vi "MRC Read.vi"(8 "error in (no error)":errorcluster, 9 "Message Data":variant, 11 "Data  in":T1={"MFC Definition"={"MFC Port"="", "MFC Enable"=TRUE, "Baud Rate"=0, "Interface type"=enum."RS-485", "Address"=0}, "Set Point Options"={"Setpoint Value"=0.0, "Mass Flow EU 2"="", "Setpoint Source"="", "Valve Mode"=""}, "Writer Queue"=refnum, "Enable"=FALSE, "Update Rate"=0, "MRC Chamber Enable"=FALSE, "Selected Gas"="", "Address String"=""} {"Set Point Options"."Setpoint Value" min=0.0 max=0.62495 format="%.5f"}) -> (0 "error out":errorcluster, 1 "Message Data Out":variant, 2 "Error Message":variant, 3 "Data out":T1={"MFC Definition"={"MFC Port"="", "MFC Enable"=TRUE, "Baud Rate"=0, "Interface type"=enum."RS-485", "Address"=0}, "Set Point Options"={"Setpoint Value"=0.0, "Mass Flow EU 2"="", "Setpoint Source"="", "Valve Mode"=""}, "Writer Queue"=refnum, "Enable"=FALSE, "Update Rate"=0, "MRC Chamber Enable"=FALSE, "Selected Gas"="", "Address String"=""} {"Set Point Options"."Setpoint Value" min=0.0 max=0.62495 format="%.5f"})   [LabVIEW 2020, in "MRC Module.lvlib"]
doc: "Perform the acquisition. Replace the contents of this diagram with calls to acquisition hardware."
uses:
  MRC Module.lvlib
  MRC Configuration.ctl
  support/Message Queue/Message Cluster.ctl
  support/Message Queue/Message Queue.lvlib
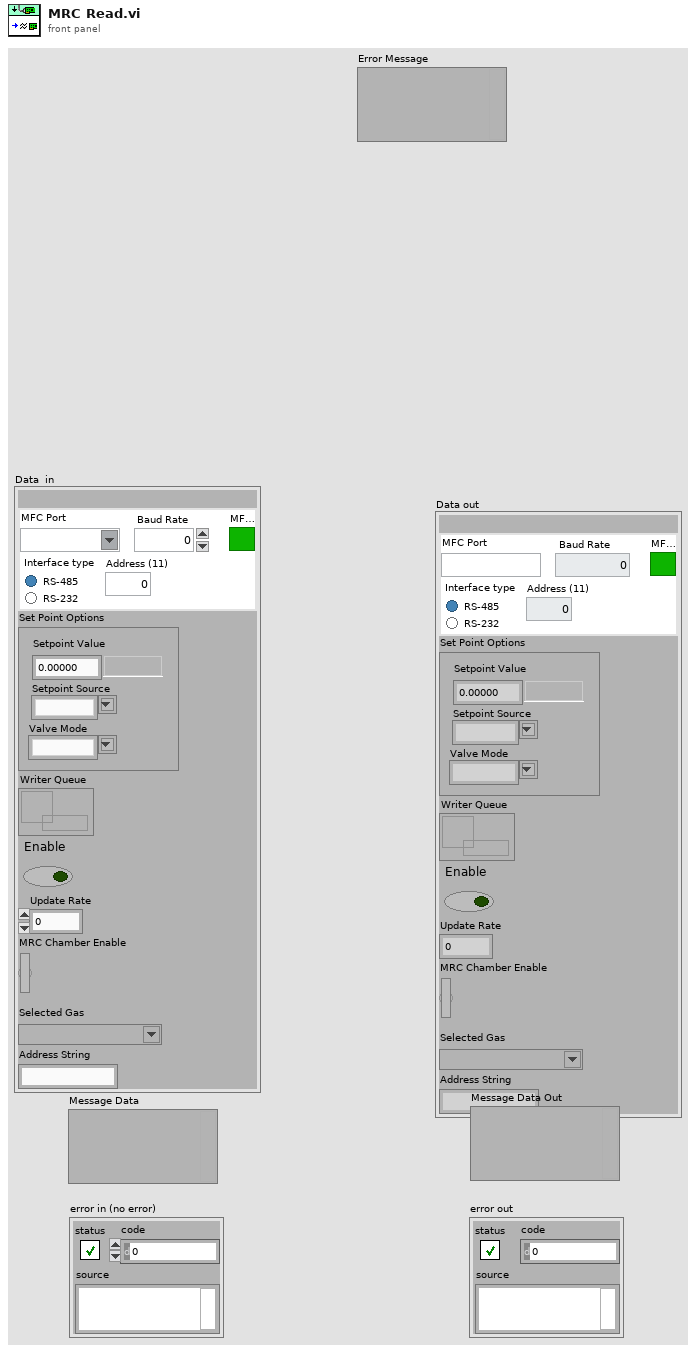
[diagram p1: front panel]
types:
  T1 = typedef "MRC Module.lvlib/MRC Configuration.ctl" = cluster{"MFC Definition":cluster{"MFC Port":refnum<visa-resource-name>, "MFC Enable":bool, "Baud Rate":i32, "Interface type":enum32{"RS-485", "RS-232"}, "Address":i32}, "Set Point Options":cluster{"Setpoint Value":dbl, "Mass Flow EU 2":string, "Setpoint Source":string, "Valve Mode":string}, "Writer Queue":refnum<queue>, "Enable":bool, "Update Rate":u32, "MRC Chamber Enable":bool, "Selected Gas":string, "Address String":string}
  T2 = typedef "Message Queue.lvlib/Message Cluster.ctl" = cluster{"Message":string, "Message Data":variant}
  T3 = cluster{"string array[0]":string, "string array[1]":string, "string array[2]":string, "string array[3]":string, "string array[4]":string, "string array[5]":string, "string array[6]":string, "string array[7]":string, "string array[8]":string, "string array[9]":string, "string array[10]":string}
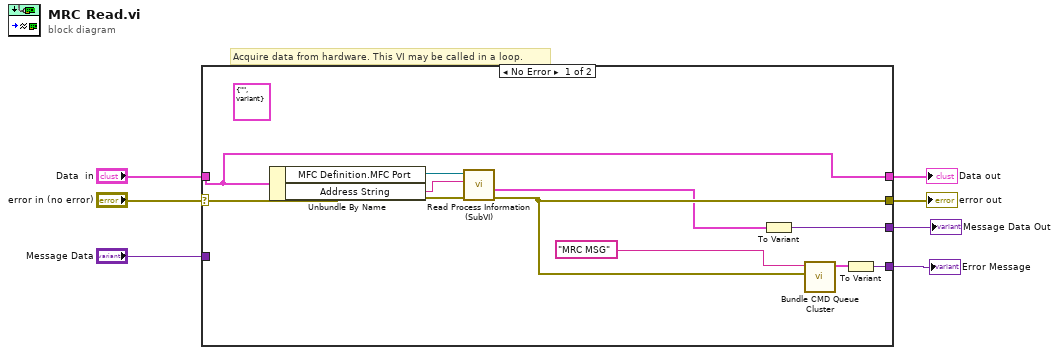
[diagram p0: block diagram]
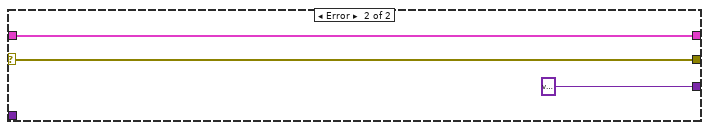
[diagram p2: hidden frame]
diagram:
  # "Acquire data from hardware. This VI may be called in a loop."
  n1 = case shown="No Error" "error in (no error)" {
    selector: "error in (no error)" -> [w11 w19]
    tunnel: [w9 w19] -> w6
    tunnel: "Data  in" -> [w14 w20]
    tunnel: [w14 w20] -> w4
    tunnel: [w13 variant ("Message Data Out")] -> w3
    tunnel: "Message Data" -> [_ _]
    tunnel: [w15 _] -> w1
    frame No Error {
      (unwired) T2 {"Message"="", "Message Data"=variant} ("element")
      n2 = Unbundle By Name(w14) -> ("MFC Definition.MFC Port"=w12:refnum<visa-resource-name>, "Address String"=w10:string)
      n3 = call "Read Process Information (SubVI).vi"("error in (no error)"=w11, "Address"=w10, "VISA Refnum in"=w12) -> ("error out"=w9:errorcluster, "PI String Array"=w8:T3)  [unwired: 4 in, 3 out]
      n4 = To Variant(anything=w8) -> (Variant=w13:variant)
      n5 = call "Bundle CMD Queue Cluster.vi"("Message Data"=w9, "Message"="MRC MSG" ("Type CMD")) -> ("Message Cluster"=w16:T2)  [unwired: 9 in]
      n6 = To Variant(anything=w16) -> (Variant=w15:variant)
    }
    frame Error {
    }
  }
  "Data out" <- w4
  "error out" <- w6
  "Message Data Out" <- w3
  "Error Message" <- w1
